vi "Autonomous Independent.vi"   [LabVIEW 2017]
doc: "This VI is called when autonomous begins, and will automatically be terminated when autonomous ends. You can carry out timed or sensor driven robot movement independently without needing to return to the caller."
uses:
  <vilib>/Rock Robotics/WPI/Utilities/WPI_GetSetVariantRefNum.vi
  <vilib>/Rock Robotics/Network Tables/NT Read Number.vi
  <vilib>/Rock Robotics/Network Tables/NT Write Numeric Array.vi
  <vilib>/Rock Robotics/Network Tables/NT Read Boolean.vi
  <vilib>/Rock Robotics/Network Tables/NT Write String.vi
  Robot Global Data.vi
  <vilib>/Rock Robotics/WPI/RobotDrive/WPI_RobotDriveArcadeDrive_Standard(NoSaturation).vi
  <vilib>/Rock Robotics/WPI/ThirdParty/Sensors/ADIS16448 IMU/ADIS16448_IMU.lvlib
panel:
  # "Be sure to right-click and choose Data Operations>>Make Current Value default if you want to save the array values with the VI"
types:
  T1 = typedef "WPI_JoystickDevRef.ctl" = cluster{"Device":T2}
  T2 = typedef "WPI_JoystickDeviceEnum.ctl" = enum16{"USB 0", "USB 1", "USB 2", "USB 3", "USB 4", "USB 5"}
  T3 = typedef "WPI_EncoderDevRef.ctl" = cluster{"DevStatus":errorcluster, "EncoderIndex":T4, "CounterIndex":T5, "DistancePerCount":dbl, "Decoding Type":T6}
  T4 = typedef "FPGA_EncoderIdx.ctl" = enum8{"Enc 0", "Enc 1", "Enc 2", "Enc 3", "Enc 4", "Enc 5", "Enc 6", "Enc 7", "Invalid"}
  T5 = typedef "FPGA_CounterCtrSystemIndex.ctl" = enum8{"Ctr 0", "Ctr 1", "Ctr 2", "Ctr 3", "Ctr 4", "Ctr 5", "Ctr 6", "Ctr 7", "Invalid"}
  T6 = typedef "WPI_EncoderType.ctl" = enum16{"1x", "2x", "4x"}
  T7 = typedef "ADIS16448_IMU.lvlib/ADI_IMU_ADIS16448_IMUDevRef.ctl" = cluster{"DevStatus":errorcluster, "Handle":i32, "SPI Bus":T8, "Device Found":bool, "Device Ready":bool, "Yaw Axis":enum16{"X", "Y", "Z"}, "AHRS Algorithm":enum16{"Complementary", "Madgwick"}, "Serial":u16, "Lot ID 2":u16, "Lot ID 1":u16, "Bytes Per Sample":u16, "Calibrate On Open?":bool}
  T8 = typedef "spi_bus.ctl" = enum16{"SPI On-Board, CS0", "SPI On-Board, CS1", "SPI On-Board, CS2", "SPI On-Board, CS3", "SPI MXP", "Invalid"}
  T9 = typedef "WPI_PotentiometerDevRef.ctl" = cluster{"DevStatus":errorcluster, "Analog Channel":T10, "Invert Output":bool}
  T10 = typedef "FPGA_AIChannel.ctl" = enum8{"AI 0", "AI 1", "AI 2", "AI 3", "AI MXP 0", "AI MXP 1", "AI MXP 2", "AI MXP 3", "Invalid"}
  T11 = typedef "WPI_RobotDriveDevRef.ctl" = cluster{"DevStatus":errorcluster, "Motors[]":T12[], "Square Inputs":bool, "Max Output":dbl}
  T12 = typedef "WPI_MotorControlDeviceRef.ctl" = cluster{"DeviceStatus":errorcluster, "Type":T13, "PWM":cluster{"PWM Channel":T14, "DeadBand":T15}, "CAN":cluster{"Device Number":u8, "SetOutput VI Ref":variant, "GetOutput VI Ref":variant, "Enable VI Ref":variant, "Disable VI Ref":variant, "Data":variant}, "Invert":bool, "DIO PWM":cluster{"PWM \"Enable\" Channel":T14, "DIOChannel":T16, "PWM Rate":dbl}}
  T13 = typedef "WPI_MotorControlType.ctl" = enum16{"PWM", "CAN", "DIO PWM"}
  T14 = typedef "FPGA_DIOPWMChannel.ctl" = enum8{"PWM 0", "PWM 1", "PWM 2", "PWM 3", "PWM 4", "PWM 5", "PWM 6", "PWM 7", "PWM 8", "PWM 9", "PWM MXP 0", "PWM MXP 1", "PWM MXP 2", "PWM MXP 3", "PWM MXP 4", "PWM MXP 5", "PWM MXP 6", "PWM MXP 7", "PWM MXP 8", "PWM MXP 9", "Invalid"}
  T15 = typedef "WPI_PWMDeadband.ctl" = cluster{"Name":string, "maxPositivePwm":i32, "minPositivePwm":i32, "centerPwm":i32, "maxNegativePwm":i32, "minNegativePwm":i32, "angularRange":u16}
  T16 = typedef "FPGA_DIOChannel.ctl" = enum8{"DIO 0", "DIO 1", "DIO 2", "DIO 3", "DIO 4", "DIO 5", "DIO 6", "DIO 7", "DIO 8", "DIO 9", "DIO MXP 0", "DIO MXP 1", "DIO MXP 2", "DIO MXP 3", "DIO MXP 4", "DIO MXP 5", "DIO MXP 6", "DIO MXP 7", "DIO MXP 8", "DIO MXP 9", "DIO MXP 10", "DIO MXP 11", "DIO MXP 12", "DIO MXP 13", "DIO MXP 14", "DIO MXP 15", "SPI Port CS1", "SPI Port CS2", "SPI Port CS3", "SPI Port MISO", "SPI Port MOSI", "Invalid"}
  T17 = cluster{"X Angle":dbl, "Y Angle":dbl, "Z Angle":dbl}
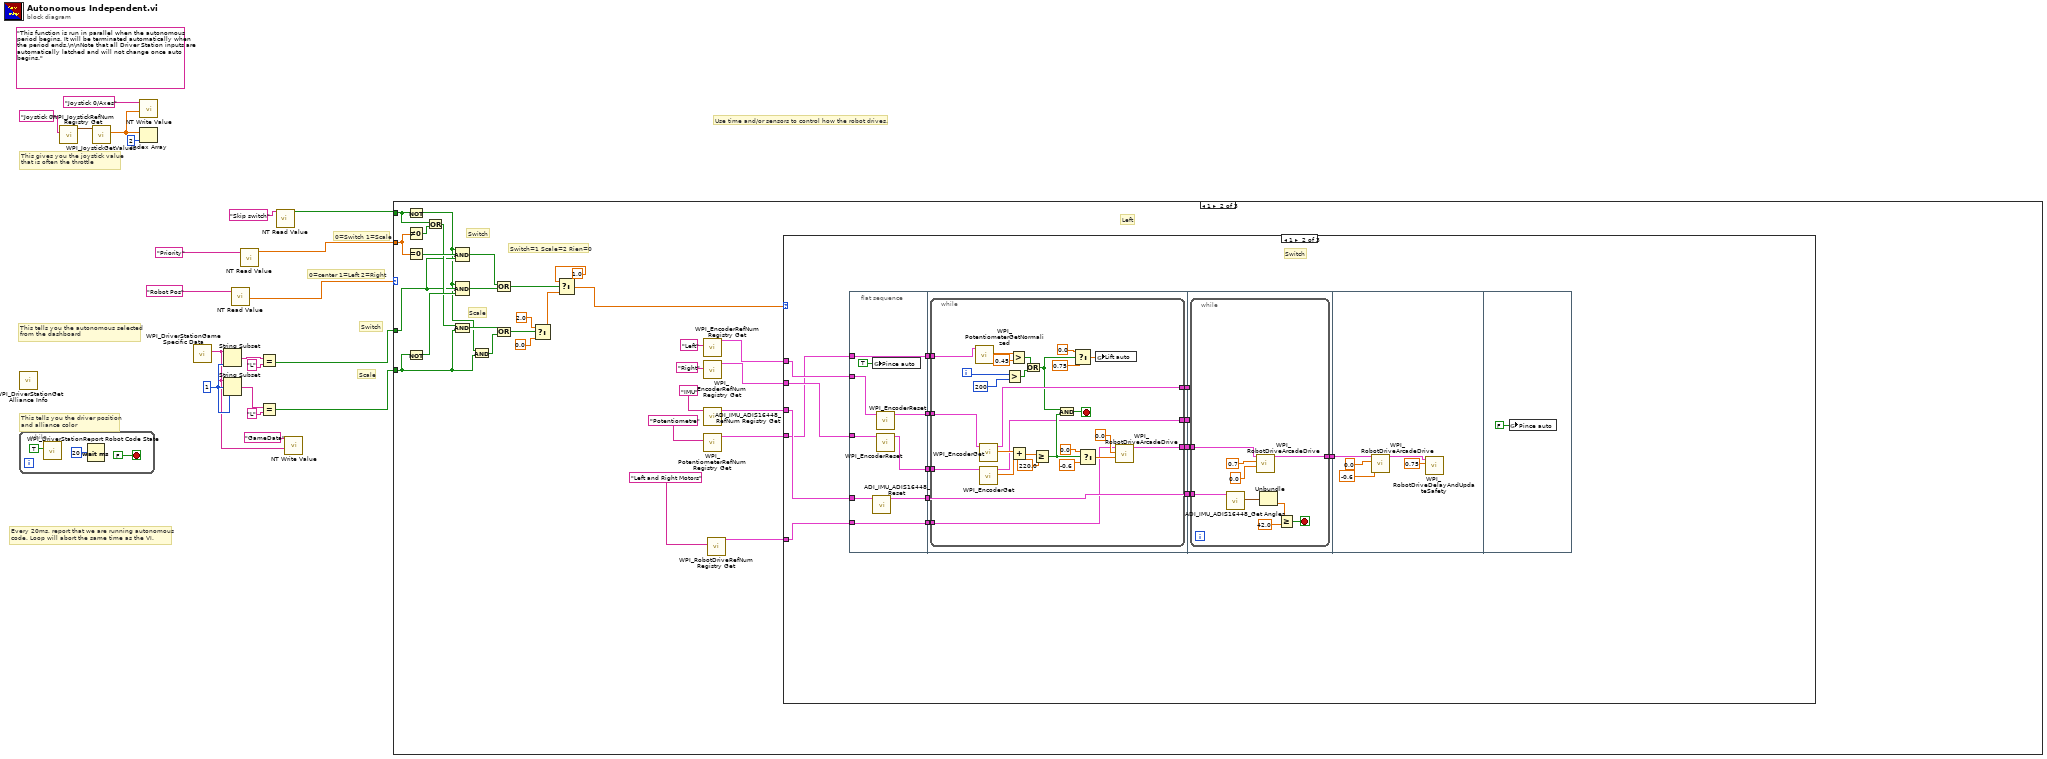
[diagram p0: block diagram]
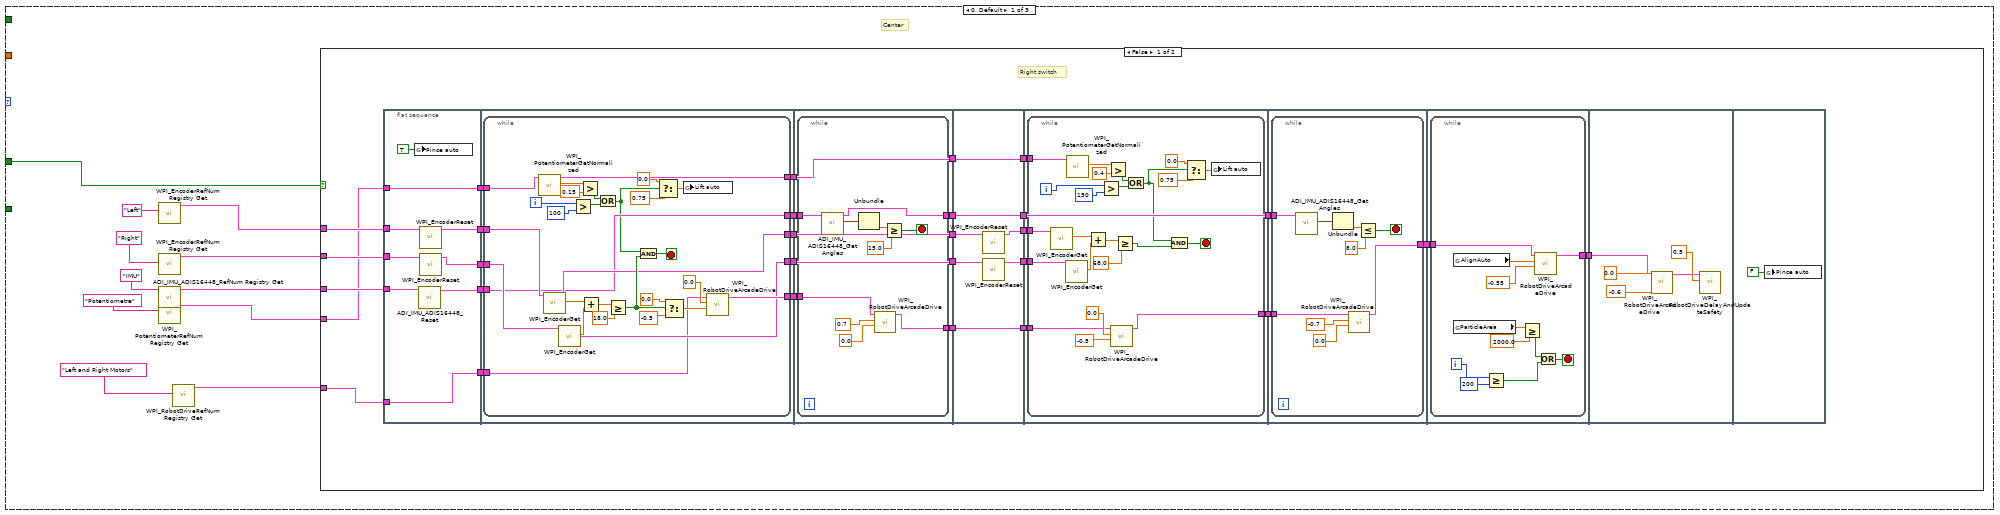
[diagram p2: hidden frame]
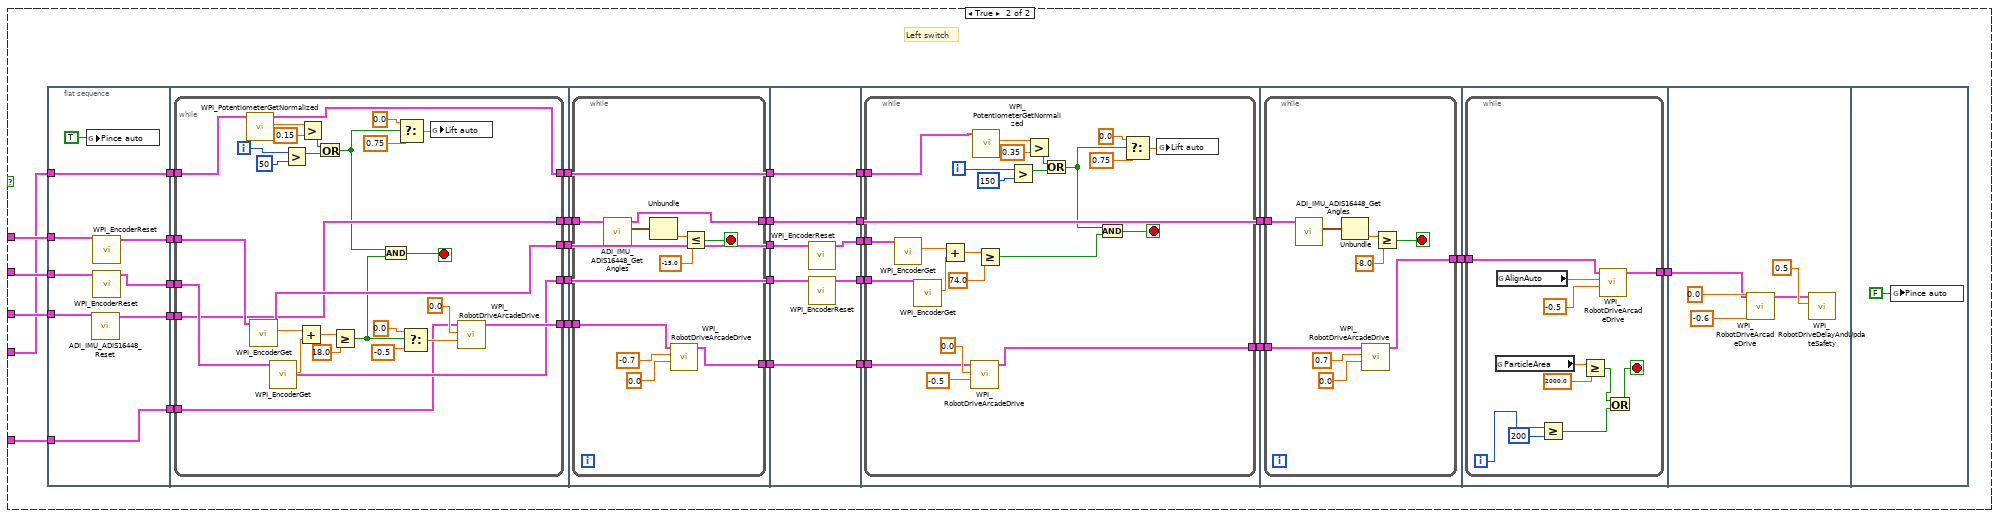
[diagram p3: hidden frame]
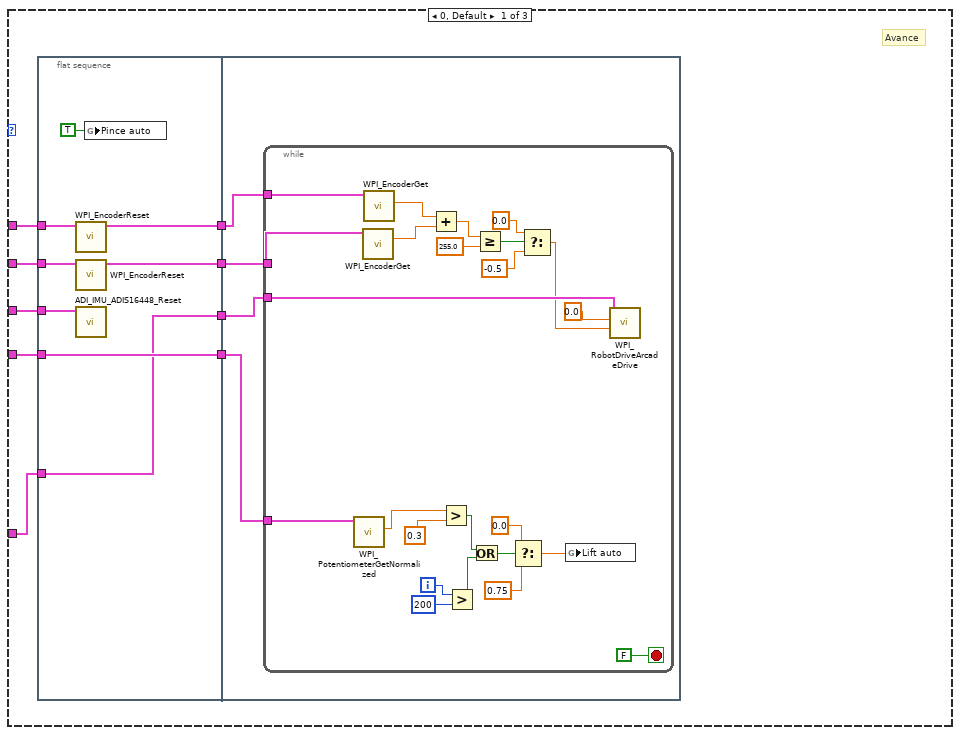
[diagram p4: hidden frame]
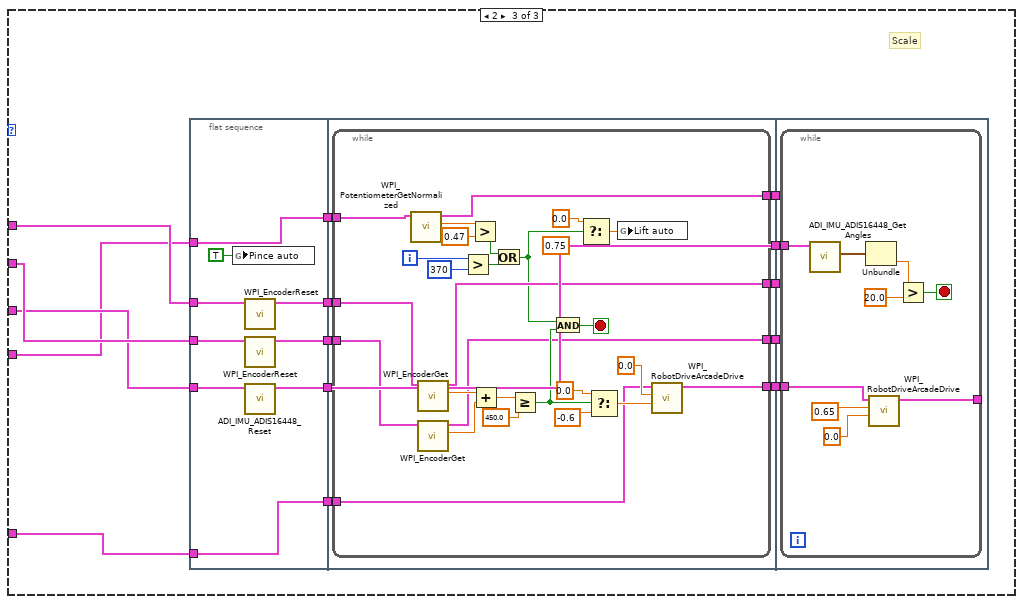
[diagram p5: hidden frame]
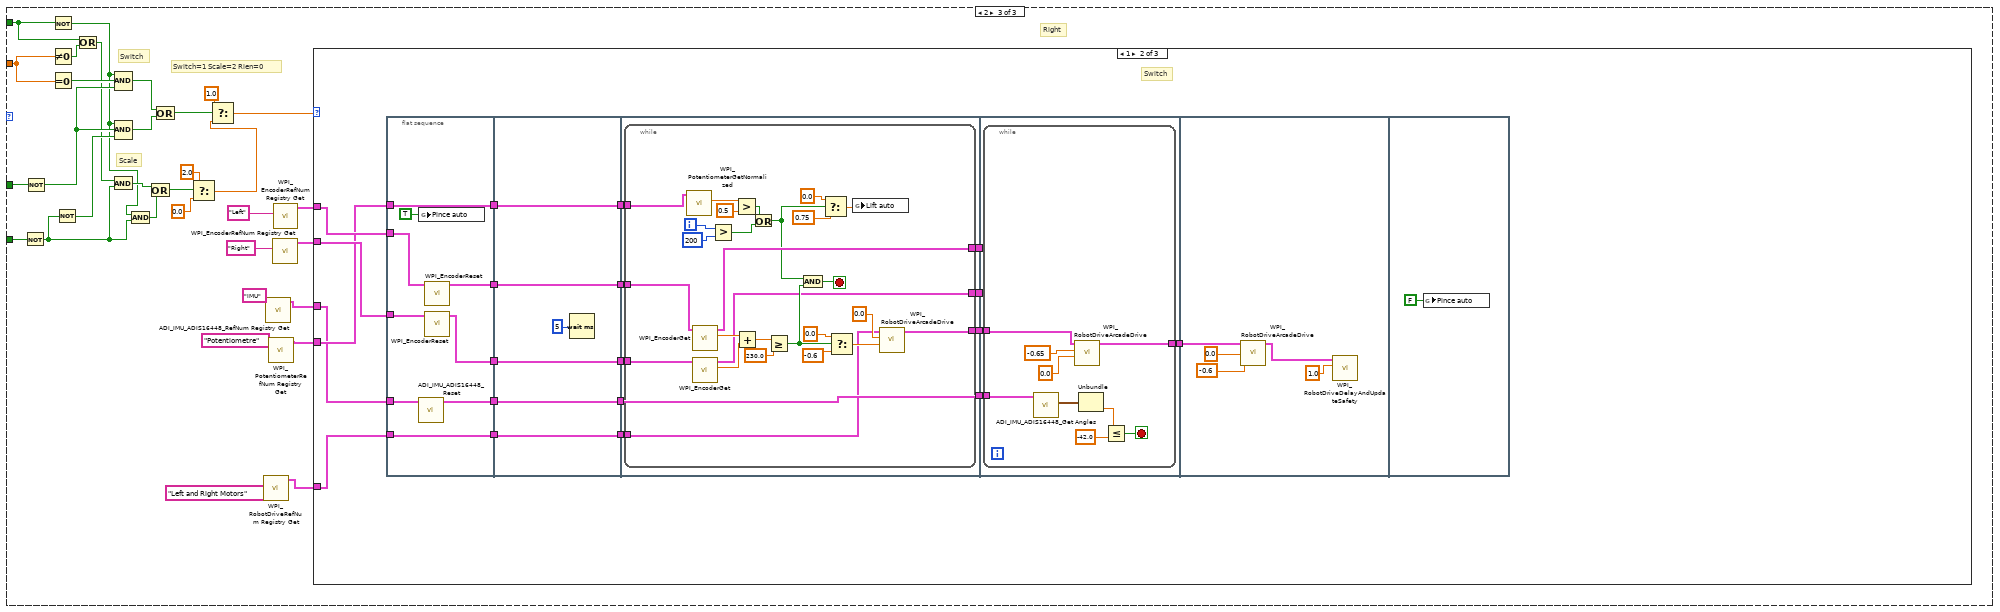
[diagram p6: hidden frame]
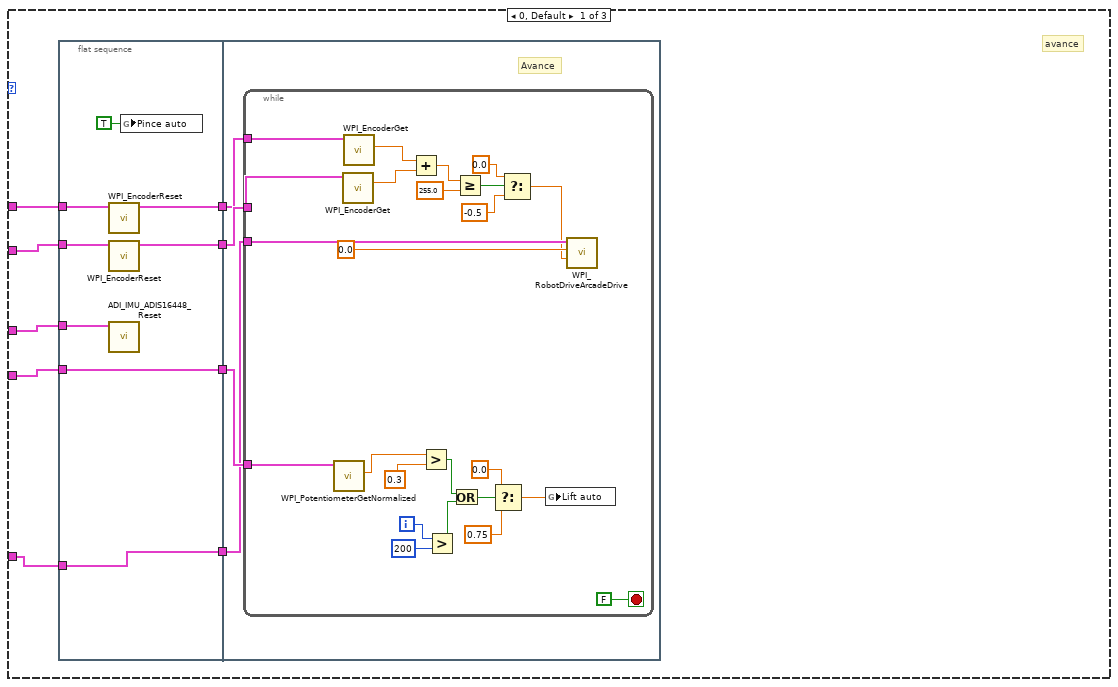
[diagram p7: hidden frame]
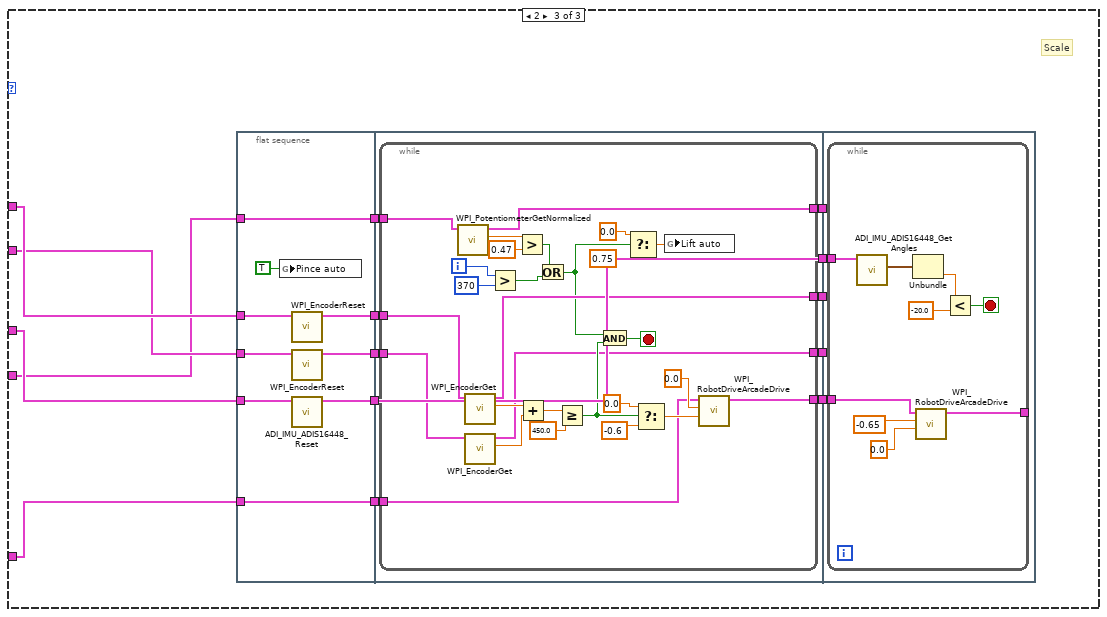
[diagram p8: hidden frame]
diagram:
  w13 = 1 ("offset (0)")
  (unwired) "This function is run in parallel when the autonomous period begins. It will be terminated automatically when the period ends.\n\nNote that all Driver Station inputs are automatically latched and will not change once auto begins."
  # "Scale"
  # "Switch"
  # "0=Switch 1=Scale"
  # "0=center 1=Left 2=Right"
  # "This tells you the autonomous selected\nfrom the dashboard"
  # "Every 20ms, report that we are running autonomous\ncode. Loop will abort the same time as the VI."
  # "This gives you the joystick value\nthat is often the throttle"
  # "Use time and/or sensors to control how the robot drives."
  # "This tells you the driver position\nand alliance color"
  n1 = while {
    stop <- FALSE stop-if-true
    n2 = call <vilib>:"WPI_DriverStationReport Robot Code State.vi"("Autonomous"=TRUE) -> ()  [unwired: 10 in, 1 out]
    n3 = Wait (ms)(milliseconds to wait=u32 20) -> ()  [unwired: 1 out]
  }
  n4 = call <vilib>:"WPI_DriverStationGet Alliance Info.vi"() -> ()  [unwired: 12 out]
  n5 = call <vilib>:"WPI_JoystickRefNum Registry Get.vi"("refnum name"="Joystick 0") -> ("JoystickDevRef"=w19:T1)  [unwired: 1 in, 9 out]
  n6 = call <vilib>:"WPI_JoystickGetValues.vi"("JoystickDevRef"=w19) -> ("Axes"=w15:dbl[])  [unwired: 6 in, 4 out]
  n7 = call-poly <vilib>:"NT Write Value.vi"("Numeric Array"=w15, "Name"="Joystick 0/Axes") -> ()  [unwired: 9 in, 1 out]
  n8 = Index Array(array=w15, index=2) -> ()  [unwired: 1 out]
  n9 = call <vilib>:"WPI_DriverStationGame Specific Data.vi"() -> ("Game Specific Data"=w2:string)  [unwired: 11 in]
  n10 = String Subset(string=w2, length (rest)=w13) -> (substring=w12:string)  [unwired: 1 in]
  n11 = String Subset(string=w2, offset (0)=w13, length (rest)=w13) -> (substring=w9:string)
  n12 = call-poly <vilib>:"NT Read Value.vi"("Name"="Robot Pos") -> ("Numeric"=w16:dbl)  [unwired: 9 in, 1 out]
  n13 = call-poly <vilib>:"NT Read Value.vi"("Name"="Priority") -> ("Numeric"=w5:dbl)  [unwired: 9 in, 1 out]
  n14 = Equal?(x=w12, y="L") -> (x = y?=w8:bool)
  n15 = Equal?(x=w9, y="L") -> (x = y?=w7:bool)
  n16 = call-poly <vilib>:"NT Read Value.vi"("Name"="Skip switch") -> ("Boolean"=w3:bool)  [unwired: 9 in, 1 out]
  n17 = call-poly <vilib>:"NT Write Value.vi"("String"=w2, "Name"="GameData") -> ()  [unwired: 9 in, 1 out]
  n18 = case shown="1" w16 {
    tunnel: w8 -> [w34 w360 w596]
    tunnel: w7 -> [_ w358 w597]
    tunnel: w5 -> [_ w372 w606]
    tunnel: w3 -> [_ w373 w607]
    frame 0, Default {
      # "Center"
      n19 = call <vilib>:"WPI_EncoderRefNum Registry Get.vi"("refnum name"="Left") -> ("EncoderDevRef"=w25:T3)  [unwired: 9 in, 1 out]
      n20 = call <vilib>:"WPI_EncoderRefNum Registry Get.vi"("refnum name"="Right") -> ("EncoderDevRef"=w26:T3)  [unwired: 9 in, 1 out]
      n21 = call <vilib>:"ADI_IMU_ADIS16448_RefNum Registry Get.vi"("refnum name"="IMU") -> ("ADI IMU DevRef"=w27:T7)  [unwired: 9 in, 1 out]
      n22 = call <vilib>:"WPI_PotentiometerRefNum Registry Get.vi"("refnum name"="Potentiometre") -> ("PotDevRef"=w28:T9)  [unwired: 9 in, 1 out]
      n23 = call <vilib>:"WPI_RobotDriveRefNum Registry Get.vi"("refnum name"="Left and Right Motors") -> ("RobotDriveDevRef"=w24:T11)  [unwired: 9 in, 1 out]
      n24 = case shown="False" w34 {
        tunnel: w28 -> [w40 w201]
        tunnel: w27 -> [w42 w203]
        tunnel: w26 -> [w43 w204]
        tunnel: w25 -> [w44 w205]
        tunnel: w24 -> [w38 w199]
        frame False {
          # "Right switch"
          n25 = flat-sequence {
            tunnel: [w71] -> w63
            tunnel: [w70] -> w62
            tunnel: [w69] -> w61
            tunnel: w44 -> [w68]
            tunnel: w43 -> [w67]
            tunnel: w42 -> [w66]
            tunnel: [w65] -> w41
            tunnel: w40 -> [w65]
            tunnel: [w64] -> w39
            tunnel: w38 -> [w64]
            tunnel: [w82] -> w60
            tunnel: [w81] -> w59
            tunnel: [w80] -> w58
            tunnel: w63 -> [w79]
            tunnel: w62 -> [w78]
            tunnel: w61 -> [w77]
            tunnel: [w76] -> w57
            tunnel: w41 -> [w75]
            tunnel: w39 -> [w74]
            tunnel: [w73] -> w35
            tunnel: [w118] -> w56
            tunnel: [w117] -> w55
            tunnel: w60 -> [w116]
            tunnel: w59 -> [w115]
            tunnel: [w115] -> w54
            tunnel: w58 -> [w114]
            tunnel: [w114] -> w53
            tunnel: w57 -> [w113]
            tunnel: [w112] -> w36
            tunnel: w35 -> [w112]
            tunnel: [w135] -> w52
            tunnel: [w134] -> w51
            tunnel: w56 -> [w133]
            tunnel: [w133] -> w50
            tunnel: [w132] -> w49
            tunnel: w55 -> [w132]
            tunnel: w54 -> [w131]
            tunnel: w53 -> [w130]
            tunnel: [w129] -> w37
            tunnel: w36 -> [w129]
            tunnel: [w141] -> w48
            tunnel: w52 -> [w140]
            tunnel: w51 -> [w139]
            tunnel: w50 -> [w138]
            tunnel: [w138] -> w47
            tunnel: w49 -> [w137]
            tunnel: w37 -> [w136]
            tunnel: [w167] -> w46
            tunnel: w48 -> [w166]
            tunnel: w47 -> [w165]
            tunnel: [w178] -> w45
            tunnel: w46 -> [w177]
            tunnel: w45 -> [w190]
            frame #0 {
              n26 = global write "Robot Global Data.vi" "Pince auto"(TRUE ("Pince auto")) -> ()
              n27 = call <vilib>:"ADI_IMU_ADIS16448_Reset.vi"("ADI IMU DevRef"=w66) -> ("ADI IMU DevRef Out"=w69:T7)  [unwired: 9 in, 1 out]
              n28 = call <vilib>:"WPI_EncoderReset.vi"("EncoderDevRef"=w68) -> ("EncoderDevRef"=w71:T3)  [unwired: 9 in, 1 out]
              n29 = call <vilib>:"WPI_EncoderReset.vi"("EncoderDevRef"=w67) -> ("EncoderDevRef"=w70:T3)  [unwired: 9 in, 1 out]
            }
            frame #1 {
              n30 = while {
                tunnel: [w96] -> w82
                tunnel: [w95] -> w81
                tunnel: [w94] -> w80
                tunnel: w79 -> [w93]
                tunnel: w78 -> [w92]
                tunnel: w77 -> [w91]
                tunnel: [w91] -> w76
                tunnel: w75 -> [w90]
                tunnel: w74 -> [w89]
                tunnel: [w83] -> w73
                i -> [w85]
                stop <- w98 stop-if-true
                n31 = call <vilib>:"WPI_PotentiometerGetNormalized.vi"("PotDevRef"=w90) -> ("Normalized Value"=w111:dbl, "PotDevRef"=w83:T9)  [unwired: 8 in, 1 out]
                n32 = call <vilib>:"WPI_EncoderGet.vi"("EncoderDevRef"=w93) -> ("Distance"=w106:dbl, "EncoderDevRef"=w94:T3)  [unwired: 5 in, 4 out]
                n33 = call <vilib>:"WPI_EncoderGet.vi"("EncoderDevRef"=w92) -> ("Distance"=w105:dbl, "EncoderDevRef"=w95:T3)  [unwired: 5 in, 4 out]
                n34 = Greater?(x=w85, y=100) -> (0:w86:bool)
                n35 = Greater?(x=w111, y=0.15) -> (0:w88:bool)
                n36 = Add(x=w106, y=w105) -> (x+y=w104:dbl)
                n37 = Or(x=w88, y=w86) -> (x .or. y?=w87:bool)
                n38 = Greater Or Equal?(x=w104, y=18.0) -> (x >= y?=w97:bool)
                n39 = And(x=w87, y=w97) -> (x .and. y?=w98:bool)
                n40 = Select(t=0.0, s=w87, f=0.75) -> (s? t:f=w107:dbl)
                n41 = Select(t=0.0, s=w97, f=-0.5) -> (s? t:f=w99:dbl)
                n42 = global write "Robot Global Data.vi" "Lift auto"(w107) -> ()
                n43 = call-poly <vilib>:"WPI_RobotDriveArcadeDrive.vi"("Y axis value"=w99, "X axis value"=0.0, "RobotDriveDevRef"=w89) -> ("RobotDriveDevRef"=w96:T11)  [unwired: 6 in, 2 out]
              }
            }
            frame #2 {
              n44 = while {
                tunnel: [w122] -> w118
                tunnel: [w121] -> w117
                tunnel: w116 -> [w120]
                tunnel: w113 -> [w119]
                stop <- w125 stop-if-true
                n45 = call <vilib>:"ADI_IMU_ADIS16448_Get Angles.vi"("ADI IMU DevRef"=w119) -> ("IMU Angles Out"=w126:T17, "ADI IMU DevRef Out"=w122:T7)  [unwired: 7 in, 2 out]
                n46 = Unbundle(w126) -> ("Z Angle"=w128:dbl)  [unwired: 2 out]
                n47 = call-poly <vilib>:"WPI_RobotDriveArcadeDrive.vi"("Y axis value"=0.0, "X axis value"=0.7, "RobotDriveDevRef"=w120) -> ("RobotDriveDevRef"=w121:T11)  [unwired: 6 in, 2 out]
                n48 = Greater Or Equal?(x=w128, y=15.0) -> (x >= y?=w125:bool)
              }
            }
            frame #3 {
              n49 = call <vilib>:"WPI_EncoderReset.vi"("EncoderDevRef"=w130) -> ("EncoderDevRef"=w135:T3)  [unwired: 9 in, 1 out]
              n50 = call <vilib>:"WPI_EncoderReset.vi"("EncoderDevRef"=w131) -> ("EncoderDevRef"=w134:T3)  [unwired: 9 in, 1 out]
            }
            frame #4 {
              n51 = while {
                tunnel: [w158] -> w141
                tunnel: w140 -> [w157]
                tunnel: w139 -> [w156]
                tunnel: w137 -> [w155]
                tunnel: w136 -> [w142]
                i -> [w143]
                stop <- w146 stop-if-true
                n52 = call <vilib>:"WPI_EncoderGet.vi"("EncoderDevRef"=w157) -> ("Distance"=w164:dbl)  [unwired: 5 in, 5 out]
                n53 = call <vilib>:"WPI_EncoderGet.vi"("EncoderDevRef"=w156) -> ("Distance"=w163:dbl)  [unwired: 5 in, 5 out]
                n54 = call <vilib>:"WPI_PotentiometerGetNormalized.vi"("PotDevRef"=w142) -> ("Normalized Value"=w154:dbl)  [unwired: 8 in, 2 out]
                n55 = Add(x=w164, y=w163) -> (x+y=w162:dbl)
                n56 = Greater?(x=w143, y=150) -> (0:w148:bool)
                n57 = Greater?(x=w154, y=0.4) -> (0:w149:bool)
                n58 = call-poly <vilib>:"WPI_RobotDriveArcadeDrive.vi"("Y axis value"=-0.5 ("f"), "X axis value"=0.0, "RobotDriveDevRef"=w155) -> ("RobotDriveDevRef"=w158:T11)  [unwired: 6 in, 2 out]
                n59 = Greater Or Equal?(x=w162, y=68.0) -> (x >= y?=w145:bool)
                n60 = Or(x=w149, y=w148) -> (x .or. y?=w144:bool)
                n61 = And(x=w144, y=w145) -> (x .and. y?=w146:bool)
                n62 = Select(t=0.0, s=w144, f=0.75) -> (s? t:f=w150:dbl)
                n63 = global write "Robot Global Data.vi" "Lift auto"(w150) -> ()
              }
            }
            frame #5 {
              n64 = while {
                tunnel: [w170] -> w167
                tunnel: w166 -> [w169]
                tunnel: w165 -> [w168]
                stop <- w173 stop-if-true
                n65 = call <vilib>:"ADI_IMU_ADIS16448_Get Angles.vi"("ADI IMU DevRef"=w168) -> ("IMU Angles Out"=w174:T17)  [unwired: 7 in, 3 out]
                n66 = Unbundle(w174) -> ("Z Angle"=w176:dbl)  [unwired: 2 out]
                n67 = call-poly <vilib>:"WPI_RobotDriveArcadeDrive.vi"("Y axis value"=0.0, "X axis value"=-0.7, "RobotDriveDevRef"=w169) -> ("RobotDriveDevRef"=w170:T11)  [unwired: 6 in, 2 out]
                n68 = Less Or Equal?(x=w176, y=8.0) -> (x <= y?=w173:bool)
              }
            }
            frame #6 {
              n69 = while {
                tunnel: [w185] -> w178
                tunnel: w177 -> [w184]
                i -> [w183]
                stop <- w181 stop-if-true
                n70 = global read "Robot Global Data.vi" "ParticleArea"() -> (w187:dbl)
                n71 = global read "Robot Global Data.vi" "AlignAuto"() -> (w189:dbl)
                n72 = Greater Or Equal?(x=w183, y=200) -> (x >= y?=w179:bool)
                n73 = Greater Or Equal?(x=w187, y=2000.0) -> (x >= y?=w180:bool)
                n74 = call-poly <vilib>:"WPI_RobotDriveArcadeDrive.vi"("Y axis value"=-0.55, "X axis value"=w189, "RobotDriveDevRef"=w184) -> ("RobotDriveDevRef"=w185:T11)  [unwired: 6 in, 2 out]
                n75 = Or(x=w180, y=w179) -> (x .or. y?=w181:bool)
              }
            }
            frame #7 {
              n76 = call-poly <vilib>:"WPI_RobotDriveArcadeDrive.vi"("Y axis value"=-0.6, "X axis value"=0.0, "RobotDriveDevRef"=w190) -> ("RobotDriveDevRef"=w191:T11)  [unwired: 6 in, 2 out]
              n77 = call <vilib>:"WPI_RobotDriveDelayAndUpdateSafety.vi"("Delay (s)"=0.5, "RobotDriveDevRef"=w191) -> ()  [unwired: 8 in, 2 out]
            }
            frame #8 {
              n78 = global write "Robot Global Data.vi" "Pince auto"(FALSE ("Pince auto")) -> ()
            }
          }
        }
        frame True {
          # "Left switch"
          n79 = flat-sequence {
            tunnel: [w232] -> w224
            tunnel: [w231] -> w223
            tunnel: [w230] -> w222
            tunnel: w205 -> [w229]
            tunnel: w204 -> [w228]
            tunnel: w203 -> [w227]
            tunnel: [w226] -> w202
            tunnel: w201 -> [w226]
            tunnel: [w225] -> w200
            tunnel: w199 -> [w225]
            tunnel: [w243] -> w221
            tunnel: [w242] -> w220
            tunnel: [w241] -> w219
            tunnel: w224 -> [w240]
            tunnel: w223 -> [w239]
            tunnel: w222 -> [w238]
            tunnel: [w237] -> w218
            tunnel: w202 -> [w236]
            tunnel: w200 -> [w235]
            tunnel: [w234] -> w198
            tunnel: [w279] -> w217
            tunnel: [w278] -> w216
            tunnel: w221 -> [w277]
            tunnel: w220 -> [w276]
            tunnel: [w276] -> w215
            tunnel: w219 -> [w275]
            tunnel: [w275] -> w214
            tunnel: w218 -> [w274]
            tunnel: w198 -> [w273]
            tunnel: [w273] -> w197
            tunnel: [w296] -> w213
            tunnel: [w295] -> w212
            tunnel: w217 -> [w294]
            tunnel: [w294] -> w211
            tunnel: [w293] -> w210
            tunnel: w216 -> [w293]
            tunnel: w215 -> [w292]
            tunnel: w214 -> [w291]
            tunnel: w197 -> [w290]
            tunnel: [w290] -> w196
            tunnel: [w302] -> w209
            tunnel: w213 -> [w301]
            tunnel: w212 -> [w300]
            tunnel: w211 -> [w299]
            tunnel: [w299] -> w208
            tunnel: w210 -> [w298]
            tunnel: w196 -> [w297]
            tunnel: [w328] -> w207
            tunnel: w209 -> [w327]
            tunnel: w208 -> [w326]
            tunnel: [w339] -> w206
            tunnel: w207 -> [w338]
            tunnel: w206 -> [w351]
            frame #0 {
              n80 = global write "Robot Global Data.vi" "Pince auto"(TRUE ("Pince auto")) -> ()
              n81 = call <vilib>:"ADI_IMU_ADIS16448_Reset.vi"("ADI IMU DevRef"=w227) -> ("ADI IMU DevRef Out"=w230:T7)  [unwired: 9 in, 1 out]
              n82 = call <vilib>:"WPI_EncoderReset.vi"("EncoderDevRef"=w229) -> ("EncoderDevRef"=w232:T3)  [unwired: 9 in, 1 out]
              n83 = call <vilib>:"WPI_EncoderReset.vi"("EncoderDevRef"=w228) -> ("EncoderDevRef"=w231:T3)  [unwired: 9 in, 1 out]
            }
            frame #1 {
              n84 = while {
                tunnel: [w264] -> w243
                tunnel: [w263] -> w242
                tunnel: [w262] -> w241
                tunnel: w240 -> [w261]
                tunnel: w239 -> [w260]
                tunnel: w238 -> [w259]
                tunnel: [w259] -> w237
                tunnel: w236 -> [w250]
                tunnel: w235 -> [w258]
                tunnel: [w249] -> w234
                i -> [w248]
                stop <- w247 stop-if-true
                n85 = call <vilib>:"WPI_PotentiometerGetNormalized.vi"("PotDevRef"=w250) -> ("Normalized Value"=w257:dbl, "PotDevRef"=w249:T9)  [unwired: 8 in, 1 out]
                n86 = call <vilib>:"WPI_EncoderGet.vi"("EncoderDevRef"=w261) -> ("Distance"=w272:dbl, "EncoderDevRef"=w262:T3)  [unwired: 5 in, 4 out]
                n87 = call <vilib>:"WPI_EncoderGet.vi"("EncoderDevRef"=w260) -> ("Distance"=w271:dbl, "EncoderDevRef"=w263:T3)  [unwired: 5 in, 4 out]
                n88 = Greater?(x=w248, y=50) -> (0:w246:bool)
                n89 = Add(x=w272, y=w271) -> (x+y=w270:dbl)
                n90 = Greater?(x=w257, y=0.15) -> (0:w252:bool)
                n91 = Or(x=w252, y=w246) -> (x .or. y?=w244:bool)
                n92 = Greater Or Equal?(x=w270, y=18.0) -> (x >= y?=w245:bool)
                n93 = And(x=w244, y=w245) -> (x .and. y?=w247:bool)
                n94 = Select(t=0.0, s=w244, f=0.75) -> (s? t:f=w253:dbl)
                n95 = Select(t=0.0, s=w245, f=-0.5) -> (s? t:f=w265:dbl)
                n96 = global write "Robot Global Data.vi" "Lift auto"(w253) -> ()
                n97 = call-poly <vilib>:"WPI_RobotDriveArcadeDrive.vi"("Y axis value"=w265, "X axis value"=0.0, "RobotDriveDevRef"=w258) -> ("RobotDriveDevRef"=w264:T11)  [unwired: 6 in, 2 out]
              }
            }
            frame #2 {
              n98 = while {
                tunnel: [w283] -> w279
                tunnel: [w282] -> w278
                tunnel: w277 -> [w281]
                tunnel: w274 -> [w280]
                stop <- w286 stop-if-true
                n99 = call <vilib>:"ADI_IMU_ADIS16448_Get Angles.vi"("ADI IMU DevRef"=w280) -> ("IMU Angles Out"=w287:T17, "ADI IMU DevRef Out"=w283:T7)  [unwired: 7 in, 2 out]
                n100 = Unbundle(w287) -> ("Z Angle"=w289:dbl)  [unwired: 2 out]
                n101 = call-poly <vilib>:"WPI_RobotDriveArcadeDrive.vi"("Y axis value"=0.0, "X axis value"=-0.7, "RobotDriveDevRef"=w281) -> ("RobotDriveDevRef"=w282:T11)  [unwired: 6 in, 2 out]
                n102 = Less Or Equal?(x=w289, y=-15.0) -> (x <= y?=w286:bool)
              }
            }
            frame #3 {
              n103 = call <vilib>:"WPI_EncoderReset.vi"("EncoderDevRef"=w291) -> ("EncoderDevRef"=w296:T3)  [unwired: 9 in, 1 out]
              n104 = call <vilib>:"WPI_EncoderReset.vi"("EncoderDevRef"=w292) -> ("EncoderDevRef"=w295:T3)  [unwired: 9 in, 1 out]
            }
            frame #4 {
              n105 = while {
                tunnel: [w319] -> w302
                tunnel: w301 -> [w318]
                tunnel: w300 -> [w317]
                tunnel: w298 -> [w316]
                tunnel: w297 -> [w304]
                i -> [w303]
                stop <- w305 stop-if-true
                n106 = call <vilib>:"WPI_EncoderGet.vi"("EncoderDevRef"=w318) -> ("Distance"=w325:dbl)  [unwired: 5 in, 5 out]
                n107 = call <vilib>:"WPI_EncoderGet.vi"("EncoderDevRef"=w317) -> ("Distance"=w324:dbl)  [unwired: 5 in, 5 out]
                n108 = Add(x=w325, y=w324) -> (x+y=w323:dbl)
                n109 = call-poly <vilib>:"WPI_RobotDriveArcadeDrive.vi"("Y axis value"=-0.5 ("f"), "X axis value"=0.0, "RobotDriveDevRef"=w316) -> ("RobotDriveDevRef"=w319:T11)  [unwired: 6 in, 2 out]
                n110 = call <vilib>:"WPI_PotentiometerGetNormalized.vi"("PotDevRef"=w304) -> ("Normalized Value"=w315:dbl)  [unwired: 8 in, 2 out]
                n111 = Greater Or Equal?(x=w323, y=74.0) -> (x >= y?=w306:bool)
                n112 = Greater?(x=w303, y=150) -> (0:w308:bool)
                n113 = Greater?(x=w315, y=0.35) -> (0:w310:bool)
                n114 = Or(x=w310, y=w308) -> (x .or. y?=w309:bool)
                n115 = And(x=w309, y=w306) -> (x .and. y?=w305:bool)
                n116 = Select(t=0.0, s=w309, f=0.75) -> (s? t:f=w311:dbl)
                n117 = global write "Robot Global Data.vi" "Lift auto"(w311) -> ()
              }
            }
            frame #5 {
              n118 = while {
                tunnel: [w331] -> w328
                tunnel: w327 -> [w330]
                tunnel: w326 -> [w329]
                stop <- w334 stop-if-true
                n119 = call <vilib>:"ADI_IMU_ADIS16448_Get Angles.vi"("ADI IMU DevRef"=w329) -> ("IMU Angles Out"=w335:T17)  [unwired: 7 in, 3 out]
                n120 = Unbundle(w335) -> ("Z Angle"=w337:dbl)  [unwired: 2 out]
                n121 = call-poly <vilib>:"WPI_RobotDriveArcadeDrive.vi"("Y axis value"=0.0, "X axis value"=0.7, "RobotDriveDevRef"=w330) -> ("RobotDriveDevRef"=w331:T11)  [unwired: 6 in, 2 out]
                n122 = Greater Or Equal?(x=w337, y=-8.0) -> (x >= y?=w334:bool)
              }
            }
            frame #6 {
              n123 = while {
                tunnel: [w346] -> w339
                tunnel: w338 -> [w345]
                i -> [w340]
                stop <- w342 stop-if-true
                n124 = global read "Robot Global Data.vi" "ParticleArea"() -> (w348:dbl)
                n125 = global read "Robot Global Data.vi" "AlignAuto"() -> (w350:dbl)
                n126 = Greater Or Equal?(x=w340, y=200) -> (x >= y?=w343:bool)
                n127 = Greater Or Equal?(x=w348, y=2000.0) -> (x >= y?=w341:bool)
                n128 = call-poly <vilib>:"WPI_RobotDriveArcadeDrive.vi"("Y axis value"=-0.5, "X axis value"=w350, "RobotDriveDevRef"=w345) -> ("RobotDriveDevRef"=w346:T11)  [unwired: 6 in, 2 out]
                n129 = Or(x=w341, y=w343) -> (x .or. y?=w342:bool)
              }
            }
            frame #7 {
              n130 = call-poly <vilib>:"WPI_RobotDriveArcadeDrive.vi"("Y axis value"=-0.6, "X axis value"=0.0, "RobotDriveDevRef"=w351) -> ("RobotDriveDevRef"=w352:T11)  [unwired: 6 in, 2 out]
              n131 = call <vilib>:"WPI_RobotDriveDelayAndUpdateSafety.vi"("Delay (s)"=0.5, "RobotDriveDevRef"=w352) -> ()  [unwired: 8 in, 2 out]
            }
            frame #8 {
              n132 = global write "Robot Global Data.vi" "Pince auto"(FALSE ("Pince auto")) -> ()
            }
          }
        }
      }
    }
    frame 1 {
      # "Switch=1 Scale=2 Rien=0"
      # "Scale"
      # "Switch"
      # "Left"
      n133 = Not(x=w373) -> (.not. x?=w357:bool)
      n134 = Not Equal To 0?(x=w372) -> (x != 0?=w381:bool)
      n135 = Equal To 0?(x=w372) -> (x = 0?=w383:bool)
      n136 = Not(x=w358) -> (.not. x?=w384:bool)
      n137 = Or(x=w373, y=w381) -> (x .or. y?=w361:bool)
      n138 = Compound Arithmetic op=AND(w357, w383, w360) -> (w386:bool)
      n139 = Compound Arithmetic op=AND(w357, w360, w384) -> (w385:bool)
      n140 = Compound Arithmetic op=AND(w361, w358) -> (w382:bool)
      n141 = And(x=w357, y=w358) -> (x .and. y?=w359:bool)
      n142 = Compound Arithmetic op=OR(w386, w385) -> (w380:bool)
      n143 = Compound Arithmetic op=OR(w382, w359) -> (w378:bool)
      n144 = Select(t=2.0, s=w378, f=0.0) -> (s? t:f=w376:dbl)
      n145 = Select(t=1.0, s=w380, f=w376) -> (s? t:f=w374:dbl)
      n146 = call <vilib>:"WPI_EncoderRefNum Registry Get.vi"("refnum name"="Left") -> ("EncoderDevRef"=w369:T3)  [unwired: 9 in, 1 out]
      n147 = call <vilib>:"WPI_EncoderRefNum Registry Get.vi"("refnum name"="Right") -> ("EncoderDevRef"=w370:T3)  [unwired: 9 in, 1 out]
      n148 = call <vilib>:"ADI_IMU_ADIS16448_RefNum Registry Get.vi"("refnum name"="IMU") -> ("ADI IMU DevRef"=w371:T7)  [unwired: 9 in, 1 out]
      n149 = call <vilib>:"WPI_PotentiometerRefNum Registry Get.vi"("refnum name"="Potentiometre") -> ("PotDevRef"=w367:T9)  [unwired: 9 in, 1 out]
      n150 = call <vilib>:"WPI_RobotDriveRefNum Registry Get.vi"("refnum name"="Left and Right Motors") -> ("RobotDriveDevRef"=w368:T11)  [unwired: 9 in, 1 out]
      n151 = case shown="1" w374 {
        tunnel: w371 -> [w395 w437 w513]
        tunnel: w370 -> [w394 w438 w514]
        tunnel: w369 -> [w393 w439 w515]
        tunnel: w368 -> [w389 w433 w509]
        tunnel: w367 -> [w392 w435 w511]
        frame 0, Default {
          # "Avance"
          n152 = flat-sequence {
            tunnel: w395 -> [w403]
            tunnel: w394 -> [w402]
            tunnel: w393 -> [w401]
            tunnel: w392 -> [w397]
            tunnel: [w400] -> w391
            tunnel: [w399] -> w390
            tunnel: w389 -> [w396]
            tunnel: [w397] -> w388
            tunnel: [w396] -> w387
            tunnel: w391 -> [w406]
            tunnel: w390 -> [w405]
            tunnel: w388 -> [w407]
            tunnel: w387 -> [w404]
            frame #0 {
              n153 = call <vilib>:"WPI_EncoderReset.vi"("EncoderDevRef"=w401) -> ("EncoderDevRef"=w400:T3)  [unwired: 9 in, 1 out]
              n154 = call <vilib>:"WPI_EncoderReset.vi"("EncoderDevRef"=w402) -> ("EncoderDevRef"=w399:T3)  [unwired: 9 in, 1 out]
              n155 = call <vilib>:"ADI_IMU_ADIS16448_Reset.vi"("ADI IMU DevRef"=w403) -> ()  [unwired: 9 in, 2 out]
              n156 = global write "Robot Global Data.vi" "Pince auto"(TRUE ("Pince auto")) -> ()
            }
            frame #1 {
              n157 = while {
                tunnel: w407 -> [w431]
                tunnel: w406 -> [w430]
                tunnel: w405 -> [w429]
                tunnel: w404 -> [w428]
                i -> [w409]
                stop <- FALSE stop-if-true
                n158 = call <vilib>:"WPI_PotentiometerGetNormalized.vi"("PotDevRef"=w431) -> ("Normalized Value"=w418:dbl)  [unwired: 8 in, 2 out]
                n159 = call <vilib>:"WPI_EncoderGet.vi"("EncoderDevRef"=w429) -> ("Distance"=w426:dbl)  [unwired: 5 in, 5 out]
                n160 = call <vilib>:"WPI_EncoderGet.vi"("EncoderDevRef"=w430) -> ("Distance"=w427:dbl)  [unwired: 5 in, 5 out]
                n161 = Add(x=w427, y=w426) -> (x+y=w425:dbl)
                n162 = Greater?(x=w418, y=0.3) -> (0:w415:bool)
                n163 = Greater?(x=w409, y=200) -> (0:w416:bool)
                n164 = Or(x=w415, y=w416) -> (x .or. y?=w414:bool)
                n165 = Greater Or Equal?(x=w425, y=255.0) -> (x >= y?=w422:bool)
                n166 = Select(t=0.0 ("Lift auto"), s=w414, f=0.75 ("Lift auto")) -> (s? t:f=w412:dbl)
                n167 = Select(t=0.0, s=w422, f=-0.5 ("Y axis value")) -> (s? t:f=w420:dbl)
                n168 = global write "Robot Global Data.vi" "Lift auto"(w412) -> ()
                n169 = call-poly <vilib>:"WPI_RobotDriveArcadeDrive.vi"("Y axis value"=w420, "X axis value"=0.0, "RobotDriveDevRef"=w428) -> ()  [unwired: 6 in, 3 out]
              }
            }
          }
        }
        frame 1 {
          # "Switch"
          n170 = flat-sequence {
            tunnel: [w454] -> w446
            tunnel: [w453] -> w445
            tunnel: [w452] -> w444
            tunnel: w439 -> [w451]
            tunnel: w438 -> [w450]
            tunnel: w437 -> [w449]
            tunnel: [w448] -> w436
            tunnel: w435 -> [w448]
            tunnel: [w447] -> w434
            tunnel: w433 -> [w447]
            tunnel: w446 -> [w463]
            tunnel: w445 -> [w462]
            tunnel: [w461] -> w443
            tunnel: w444 -> [w461]
            tunnel: [w460] -> w442
            tunnel: [w459] -> w441
            tunnel: [w458] -> w440
            tunnel: w436 -> [w457]
            tunnel: w434 -> [w456]
            tunnel: w443 -> [w493]
            tunnel: w442 -> [w492]
            tunnel: w441 -> [_]
            tunnel: w440 -> [_]
            tunnel: [w491] -> w432
            tunnel: w432 -> [w507]
            frame #0 {
              n171 = global write "Robot Global Data.vi" "Pince auto"(TRUE ("Pince auto")) -> ()
              n172 = call <vilib>:"ADI_IMU_ADIS16448_Reset.vi"("ADI IMU DevRef"=w449) -> ("ADI IMU DevRef Out"=w452:T7)  [unwired: 9 in, 1 out]
              n173 = call <vilib>:"WPI_EncoderReset.vi"("EncoderDevRef"=w451) -> ("EncoderDevRef"=w454:T3)  [unwired: 9 in, 1 out]
              n174 = call <vilib>:"WPI_EncoderReset.vi"("EncoderDevRef"=w450) -> ("EncoderDevRef"=w453:T3)  [unwired: 9 in, 1 out]
            }
            frame #1 {
              n175 = while {
                tunnel: w463 -> [w475]
                tunnel: w462 -> [w474]
                tunnel: [w473] -> w459
                tunnel: [w472] -> w458
                tunnel: [w471] -> w460
                tunnel: w457 -> [w470]
                tunnel: w456 -> [w469]
                i -> [w468]
                stop <- w477 stop-if-true
                n176 = call <vilib>:"WPI_PotentiometerGetNormalized.vi"("PotDevRef"=w470) -> ("Normalized Value"=w490:dbl)  [unwired: 8 in, 2 out]
                n177 = call <vilib>:"WPI_EncoderGet.vi"("EncoderDevRef"=w475) -> ("Distance"=w485:dbl, "EncoderDevRef"=w473:T3)  [unwired: 5 in, 4 out]
                n178 = call <vilib>:"WPI_EncoderGet.vi"("EncoderDevRef"=w474) -> ("Distance"=w484:dbl, "EncoderDevRef"=w472:T3)  [unwired: 5 in, 4 out]
                n179 = Greater?(x=w468, y=200) -> (0:w464:bool)
                n180 = Greater?(x=w490, y=0.45) -> (0:w466:bool)
                n181 = Add(x=w485, y=w484) -> (x+y=w483:dbl)
                n182 = Or(x=w466, y=w464) -> (x .or. y?=w465:bool)
                n183 = Greater Or Equal?(x=w483, y=220.0) -> (x >= y?=w476:bool)
                n184 = And(x=w465, y=w476) -> (x .and. y?=w477:bool)
                n185 = Select(t=0.0, s=w465, f=0.75) -> (s? t:f=w486:dbl)
                n186 = Select(t=0.0, s=w476, f=-0.6) -> (s? t:f=w478:dbl)
                n187 = global write "Robot Global Data.vi" "Lift auto"(w486) -> ()
                n188 = call-poly <vilib>:"WPI_RobotDriveArcadeDrive.vi"("Y axis value"=w478, "X axis value"=0.0, "RobotDriveDevRef"=w469) -> ("RobotDriveDevRef"=w471:T11)  [unwired: 6 in, 2 out]
              }
            }
            frame #2 {
              n189 = while {
                tunnel: w493 -> [w498]
                tunnel: w492 -> [w495]
                tunnel: [w494] -> w491
                stop <- w499 stop-if-true
                n190 = call <vilib>:"ADI_IMU_ADIS16448_Get Angles.vi"("ADI IMU DevRef"=w498) -> ("IMU Angles Out"=w502:T17)  [unwired: 7 in, 3 out]
                n191 = call-poly <vilib>:"WPI_RobotDriveArcadeDrive.vi"("Y axis value"=0.0, "X axis value"=0.7, "RobotDriveDevRef"=w495) -> ("RobotDriveDevRef"=w494:T11)  [unwired: 6 in, 2 out]
                n192 = Unbundle(w502) -> ("Z Angle"=w501:dbl)  [unwired: 2 out]
                n193 = Greater Or Equal?(x=w501, y=42.0) -> (x >= y?=w499:bool)
              }
            }
            frame #3 {
              n194 = call-poly <vilib>:"WPI_RobotDriveArcadeDrive.vi"("Y axis value"=-0.6, "X axis value"=0.0, "RobotDriveDevRef"=w507) -> ("RobotDriveDevRef"=w504:T11)  [unwired: 6 in, 2 out]
              n195 = call <vilib>:"WPI_RobotDriveDelayAndUpdateSafety.vi"("Delay (s)"=0.75, "RobotDriveDevRef"=w504) -> ()  [unwired: 8 in, 2 out]
            }
            frame #4 {
              n196 = global write "Robot Global Data.vi" "Pince auto"(FALSE ("Pince auto")) -> ()
            }
          }
        }
        frame 2 {
          # "Scale"
          n197 = flat-sequence {
            tunnel: [w531] -> w523
            tunnel: [w530] -> w522
            tunnel: [w529] -> w521
            tunnel: w515 -> [w528]
            tunnel: w514 -> [w527]
            tunnel: w513 -> [w526]
            tunnel: [w525] -> w512
            tunnel: w511 -> [w525]
            tunnel: [w524] -> w510
            tunnel: w509 -> [w524]
            tunnel: w523 -> [w541]
            tunnel: w522 -> [w540]
            tunnel: [w539] -> w520
            tunnel: w521 -> [w538]
            tunnel: [w538] -> w519
            tunnel: [w537] -> w518
            tunnel: [w536] -> w517
            tunnel: [w535] -> w516
            tunnel: w512 -> [w534]
            tunnel: w510 -> [w533]
            tunnel: w520 -> [w571]
            tunnel: w519 -> [w570]
            tunnel: w518 -> [_]
            tunnel: w517 -> [_]
            tunnel: w516 -> [_]
            frame #0 {
              n198 = global write "Robot Global Data.vi" "Pince auto"(TRUE ("Pince auto")) -> ()
              n199 = call <vilib>:"WPI_EncoderReset.vi"("EncoderDevRef"=w528) -> ("EncoderDevRef"=w531:T3)  [unwired: 9 in, 1 out]
              n200 = call <vilib>:"WPI_EncoderReset.vi"("EncoderDevRef"=w527) -> ("EncoderDevRef"=w530:T3)  [unwired: 9 in, 1 out]
              n201 = call <vilib>:"ADI_IMU_ADIS16448_Reset.vi"("ADI IMU DevRef"=w526) -> ("ADI IMU DevRef Out"=w529:T7)  [unwired: 9 in, 1 out]
            }
            frame #1 {
              n202 = while {
                tunnel: [w554] -> w536
                tunnel: [w553] -> w535
                tunnel: [w552] -> w539
                tunnel: w541 -> [w551]
                tunnel: w540 -> [w550]
                tunnel: [w549] -> w537
                tunnel: w534 -> [w548]
                tunnel: w533 -> [w547]
                i -> [w543]
                stop <- w556 stop-if-true
                n203 = call <vilib>:"WPI_PotentiometerGetNormalized.vi"("PotDevRef"=w548) -> ("Normalized Value"=w569:dbl, "PotDevRef"=w549:T9)  [unwired: 8 in, 1 out]
                n204 = call <vilib>:"WPI_EncoderGet.vi"("EncoderDevRef"=w551) -> ("Distance"=w564:dbl, "EncoderDevRef"=w554:T3)  [unwired: 5 in, 4 out]
                n205 = call <vilib>:"WPI_EncoderGet.vi"("EncoderDevRef"=w550) -> ("Distance"=w563:dbl, "EncoderDevRef"=w553:T3)  [unwired: 5 in, 4 out]
                n206 = Greater?(x=w543, y=370) -> (0:w544:bool)
                n207 = Greater?(x=w569, y=0.47) -> (0:w546:bool)
                n208 = Add(x=w564, y=w563) -> (x+y=w562:dbl)
                n209 = Or(x=w546, y=w544) -> (x .or. y?=w545:bool)
                n210 = Greater Or Equal?(x=w562, y=450.0) -> (x >= y?=w555:bool)
                n211 = And(x=w545, y=w555) -> (x .and. y?=w556:bool)
                n212 = Select(t=0.0, s=w545, f=0.75) -> (s? t:f=w565:dbl)
                n213 = Select(t=0.0, s=w555, f=-0.6) -> (s? t:f=w557:dbl)
                n214 = global write "Robot Global Data.vi" "Lift auto"(w565) -> ()
                n215 = call-poly <vilib>:"WPI_RobotDriveArcadeDrive.vi"("Y axis value"=w557, "X axis value"=0.0, "RobotDriveDevRef"=w547) -> ("RobotDriveDevRef"=w552:T11)  [unwired: 6 in, 2 out]
              }
            }
            frame #2 {
              n216 = while {
                tunnel: w571 -> [w574]
                tunnel: w570 -> [w573]
                tunnel: [w572] -> _
                stop <- w577 stop-if-true
                n217 = call <vilib>:"ADI_IMU_ADIS16448_Get Angles.vi"("ADI IMU DevRef"=w573) -> ("IMU Angles Out"=w580:T17)  [unwired: 7 in, 3 out]
                n218 = Unbundle(w580) -> ("Z Angle"=w579:dbl)  [unwired: 2 out]
                n219 = call-poly <vilib>:"WPI_RobotDriveArcadeDrive.vi"("Y axis value"=0.0, "X axis value"=0.65, "RobotDriveDevRef"=w574) -> ("RobotDriveDevRef"=w572:T11)  [unwired: 6 in, 2 out]
                n220 = Greater?(x=w579, y=20.0) -> (0:w577:bool)
              }
            }
          }
        }
      }
    }
    frame 2 {
      # "Switch=1 Scale=2 Rien=0"
      # "Scale"
      # "Switch"
      # "Right"
      n221 = Not(x=w597) -> (.not. x?=w582:bool)
      n222 = Not(x=w596) -> (.not. x?=w585:bool)
      n223 = Not(x=w607) -> (.not. x?=w581:bool)
      n224 = Not Equal To 0?(x=w606) -> (x != 0?=w605:bool)
      n225 = Equal To 0?(x=w606) -> (x = 0?=w609:bool)
      n226 = Not(x=w582) -> (.not. x?=w610:bool)
      n227 = Or(x=w607, y=w605) -> (x .or. y?=w584:bool)
      n228 = Compound Arithmetic op=AND(w581, w609, w585) -> (w612:bool)
      n229 = Compound Arithmetic op=AND(w581, w585, w610) -> (w611:bool)
      n230 = Compound Arithmetic op=AND(w584, w582) -> (w608:bool)
      n231 = And(x=w581, y=w582) -> (x .and. y?=w583:bool)
      n232 = Compound Arithmetic op=OR(w608, w583) -> (w602:bool)
      n233 = Compound Arithmetic op=OR(w612, w611) -> (w604:bool)
      n234 = Select(t=2.0, s=w602, f=0.0) -> (s? t:f=w600:dbl)
      n235 = Select(t=1.0, s=w604, f=w600) -> (s? t:f=w598:dbl)
      n236 = call <vilib>:"WPI_RobotDriveRefNum Registry Get.vi"("refnum name"="Left and Right Motors") -> ("RobotDriveDevRef"=w586:T11)  [unwired: 9 in, 1 out]
      n237 = call <vilib>:"ADI_IMU_ADIS16448_RefNum Registry Get.vi"("refnum name"="IMU") -> ("ADI IMU DevRef"=w588:T7)  [unwired: 9 in, 1 out]
      n238 = call <vilib>:"WPI_PotentiometerRefNum Registry Get.vi"("refnum name"="Potentiometre") -> ("PotDevRef"=w587:T9)  [unwired: 9 in, 1 out]
      n239 = call <vilib>:"WPI_EncoderRefNum Registry Get.vi"("refnum name"="Right") -> ("EncoderDevRef"=w589:T3)  [unwired: 9 in, 1 out]
      n240 = call <vilib>:"WPI_EncoderRefNum Registry Get.vi"("refnum name"="Left") -> ("EncoderDevRef"=w590:T3)  [unwired: 9 in, 1 out]
      n241 = case shown="1" w598 {
        tunnel: w590 -> [w619 w673 w752]
        tunnel: w589 -> [w618 w672 w751]
        tunnel: w588 -> [w617 w670 w750]
        tunnel: w587 -> [w616 w671 w748]
        tunnel: w586 -> [w614 w669 w746]
        frame 0, Default {
          # "avance"
          # "Avance"
          n242 = flat-sequence {
            tunnel: w617 -> [w629]
            tunnel: w618 -> [w628]
            tunnel: w619 -> [w627]
            tunnel: w616 -> [w623]
            tunnel: [w626] -> w621
            tunnel: [w625] -> w620
            tunnel: [w623] -> w615
            tunnel: w614 -> [w622]
            tunnel: [w622] -> w613
            tunnel: w621 -> [w630]
            tunnel: w620 -> [w631]
            tunnel: w615 -> [w633]
            tunnel: w613 -> [w632]
            frame #0 {
              n243 = call <vilib>:"WPI_EncoderReset.vi"("EncoderDevRef"=w627) -> ("EncoderDevRef"=w626:T3)  [unwired: 9 in, 1 out]
              n244 = call <vilib>:"WPI_EncoderReset.vi"("EncoderDevRef"=w628) -> ("EncoderDevRef"=w625:T3)  [unwired: 9 in, 1 out]
              n245 = call <vilib>:"ADI_IMU_ADIS16448_Reset.vi"("ADI IMU DevRef"=w629) -> ()  [unwired: 9 in, 2 out]
              n246 = global write "Robot Global Data.vi" "Pince auto"(TRUE ("Pince auto")) -> ()
            }
            frame #1 {
              n247 = while {
                tunnel: w633 -> [w657]
                tunnel: w630 -> [w656]
                tunnel: w631 -> [w655]
                tunnel: w632 -> [w654]
                i -> [w635]
                stop <- FALSE stop-if-true
                n248 = call <vilib>:"WPI_PotentiometerGetNormalized.vi"("PotDevRef"=w657) -> ("Normalized Value"=w644:dbl)  [unwired: 8 in, 2 out]
                n249 = call <vilib>:"WPI_EncoderGet.vi"("EncoderDevRef"=w655) -> ("Distance"=w652:dbl)  [unwired: 5 in, 5 out]
                n250 = call <vilib>:"WPI_EncoderGet.vi"("EncoderDevRef"=w656) -> ("Distance"=w653:dbl)  [unwired: 5 in, 5 out]
                n251 = Add(x=w653, y=w652) -> (x+y=w651:dbl)
                n252 = Greater?(x=w644, y=0.3) -> (0:w641:bool)
                n253 = Greater?(x=w635, y=200) -> (0:w642:bool)
                n254 = Or(x=w641, y=w642) -> (x .or. y?=w640:bool)
                n255 = Greater Or Equal?(x=w651, y=255.0) -> (x >= y?=w648:bool)
                n256 = Select(t=0.0 ("Lift auto"), s=w640, f=0.75 ("Lift auto")) -> (s? t:f=w638:dbl)
                n257 = Select(t=0.0, s=w648, f=-0.5 ("Y axis value")) -> (s? t:f=w646:dbl)
                n258 = global write "Robot Global Data.vi" "Lift auto"(w638) -> ()
                n259 = call-poly <vilib>:"WPI_RobotDriveArcadeDrive.vi"("Y axis value"=w646, "X axis value"=0.0, "RobotDriveDevRef"=w654) -> ()  [unwired: 6 in, 3 out]
              }
            }
          }
        }
        frame 1 {
          # "Switch"
          n260 = flat-sequence {
            tunnel: [w685] -> w668
            tunnel: [w684] -> w666
            tunnel: [w683] -> w664
            tunnel: w673 -> [w682]
            tunnel: w672 -> [w681]
            tunnel: w670 -> [w680]
            tunnel: [w679] -> w662
            tunnel: w671 -> [w679]
            tunnel: [w678] -> w660
            tunnel: w669 -> [w678]
            tunnel: w668 -> [w692]
            tunnel: [w692] -> w667
            tunnel: w666 -> [w691]
            tunnel: [w691] -> w665
            tunnel: w664 -> [w690]
            tunnel: [w690] -> w663
            tunnel: w662 -> [w689]
            tunnel: [w689] -> w661
            tunnel: w660 -> [w688]
            tunnel: [w688] -> w659
            tunnel: w667 -> [w700]
            tunnel: w665 -> [w699]
            tunnel: [w698] -> w677
            tunnel: w663 -> [w698]
            tunnel: [w697] -> w676
            tunnel: [w696] -> w675
            tunnel: [w695] -> w674
            tunnel: w661 -> [w694]
            tunnel: w659 -> [w693]
            tunnel: w677 -> [w730]
            tunnel: w676 -> [w729]
            tunnel: w675 -> [_]
            tunnel: w674 -> [_]
            tunnel: [w728] -> w658
            tunnel: w658 -> [w744]
            frame #0 {
              n261 = global write "Robot Global Data.vi" "Pince auto"(TRUE ("Pince auto")) -> ()
              n262 = call <vilib>:"ADI_IMU_ADIS16448_Reset.vi"("ADI IMU DevRef"=w680) -> ("ADI IMU DevRef Out"=w683:T7)  [unwired: 9 in, 1 out]
              n263 = call <vilib>:"WPI_EncoderReset.vi"("EncoderDevRef"=w682) -> ("EncoderDevRef"=w685:T3)  [unwired: 9 in, 1 out]
              n264 = call <vilib>:"WPI_EncoderReset.vi"("EncoderDevRef"=w681) -> ("EncoderDevRef"=w684:T3)  [unwired: 9 in, 1 out]
            }
            frame #1 {
              n265 = Wait (ms)(milliseconds to wait=u32 5) -> ()  [unwired: 1 out]
            }
            frame #2 {
              n266 = while {
                tunnel: w700 -> [w712]
                tunnel: w699 -> [w711]
                tunnel: [w710] -> w696
                tunnel: [w709] -> w695
                tunnel: [w708] -> w697
                tunnel: w694 -> [w707]
                tunnel: w693 -> [w706]
                i -> [w702]
                stop <- w714 stop-if-true
                n267 = call <vilib>:"WPI_PotentiometerGetNormalized.vi"("PotDevRef"=w707) -> ("Normalized Value"=w727:dbl)  [unwired: 8 in, 2 out]
                n268 = call <vilib>:"WPI_EncoderGet.vi"("EncoderDevRef"=w712) -> ("Distance"=w722:dbl, "EncoderDevRef"=w710:T3)  [unwired: 5 in, 4 out]
                n269 = call <vilib>:"WPI_EncoderGet.vi"("EncoderDevRef"=w711) -> ("Distance"=w721:dbl, "EncoderDevRef"=w709:T3)  [unwired: 5 in, 4 out]
                n270 = Greater?(x=w702, y=200) -> (0:w703:bool)
                n271 = Greater?(x=w727, y=0.5) -> (0:w704:bool)
                n272 = Add(x=w722, y=w721) -> (x+y=w720:dbl)
                n273 = Or(x=w704, y=w703) -> (x .or. y?=w705:bool)
                n274 = Greater Or Equal?(x=w720, y=230.0) -> (x >= y?=w713:bool)
                n275 = And(x=w705, y=w713) -> (x .and. y?=w714:bool)
                n276 = Select(t=0.0, s=w705, f=0.75) -> (s? t:f=w723:dbl)
                n277 = Select(t=0.0, s=w713, f=-0.6) -> (s? t:f=w715:dbl)
                n278 = global write "Robot Global Data.vi" "Lift auto"(w723) -> ()
                n279 = call-poly <vilib>:"WPI_RobotDriveArcadeDrive.vi"("Y axis value"=w715, "X axis value"=0.0, "RobotDriveDevRef"=w706) -> ("RobotDriveDevRef"=w708:T11)  [unwired: 6 in, 2 out]
              }
            }
            frame #3 {
              n280 = while {
                tunnel: w730 -> [w735]
                tunnel: w729 -> [w732]
                tunnel: [w731] -> w728
                stop <- w736 stop-if-true
                n281 = call <vilib>:"ADI_IMU_ADIS16448_Get Angles.vi"("ADI IMU DevRef"=w735) -> ("IMU Angles Out"=w739:T17)  [unwired: 7 in, 3 out]
                n282 = call-poly <vilib>:"WPI_RobotDriveArcadeDrive.vi"("Y axis value"=0.0, "X axis value"=-0.65, "RobotDriveDevRef"=w732) -> ("RobotDriveDevRef"=w731:T11)  [unwired: 6 in, 2 out]
                n283 = Unbundle(w739) -> ("Z Angle"=w738:dbl)  [unwired: 2 out]
                n284 = Less Or Equal?(x=w738, y=-42.0) -> (x <= y?=w736:bool)
              }
            }
            frame #4 {
              n285 = call-poly <vilib>:"WPI_RobotDriveArcadeDrive.vi"("Y axis value"=-0.6, "X axis value"=0.0, "RobotDriveDevRef"=w744) -> ("RobotDriveDevRef"=w740:T11)  [unwired: 6 in, 2 out]
              n286 = call <vilib>:"WPI_RobotDriveDelayAndUpdateSafety.vi"("Delay (s)"=1.0, "RobotDriveDevRef"=w740) -> ()  [unwired: 8 in, 2 out]
            }
            frame #5 {
              n287 = global write "Robot Global Data.vi" "Pince auto"(FALSE ("Pince auto")) -> ()
            }
          }
        }
        frame 2 {
          # "Scale"
          n288 = flat-sequence {
            tunnel: [w768] -> w760
            tunnel: [w767] -> w759
            tunnel: [w766] -> w758
            tunnel: w752 -> [w765]
            tunnel: w751 -> [w764]
            tunnel: w750 -> [w763]
            tunnel: [w762] -> w749
            tunnel: w748 -> [w762]
            tunnel: [w761] -> w747
            tunnel: w746 -> [w761]
            tunnel: w760 -> [w778]
            tunnel: w759 -> [w777]
            tunnel: [w776] -> w757
            tunnel: w758 -> [w775]
            tunnel: [w775] -> w756
            tunnel: [w774] -> w755
            tunnel: [w773] -> w754
            tunnel: [w772] -> w753
            tunnel: w749 -> [w771]
            tunnel: w747 -> [w770]
            tunnel: w757 -> [w808]
            tunnel: w756 -> [w807]
            tunnel: w755 -> [_]
            tunnel: w754 -> [_]
            tunnel: w753 -> [_]
            frame #0 {
              n289 = global write "Robot Global Data.vi" "Pince auto"(TRUE ("Pince auto")) -> ()
              n290 = call <vilib>:"WPI_EncoderReset.vi"("EncoderDevRef"=w765) -> ("EncoderDevRef"=w768:T3)  [unwired: 9 in, 1 out]
              n291 = call <vilib>:"WPI_EncoderReset.vi"("EncoderDevRef"=w764) -> ("EncoderDevRef"=w767:T3)  [unwired: 9 in, 1 out]
              n292 = call <vilib>:"ADI_IMU_ADIS16448_Reset.vi"("ADI IMU DevRef"=w763) -> ("ADI IMU DevRef Out"=w766:T7)  [unwired: 9 in, 1 out]
            }
            frame #1 {
              n293 = while {
                tunnel: [w791] -> w773
                tunnel: [w790] -> w772
                tunnel: [w789] -> w776
                tunnel: w778 -> [w788]
                tunnel: w777 -> [w787]
                tunnel: [w786] -> w774
                tunnel: w771 -> [w785]
                tunnel: w770 -> [w784]
                i -> [w783]
                stop <- w793 stop-if-true
                n294 = call <vilib>:"WPI_PotentiometerGetNormalized.vi"("PotDevRef"=w785) -> ("Normalized Value"=w806:dbl, "PotDevRef"=w786:T9)  [unwired: 8 in, 1 out]
                n295 = call <vilib>:"WPI_EncoderGet.vi"("EncoderDevRef"=w788) -> ("Distance"=w801:dbl, "EncoderDevRef"=w791:T3)  [unwired: 5 in, 4 out]
                n296 = call <vilib>:"WPI_EncoderGet.vi"("EncoderDevRef"=w787) -> ("Distance"=w800:dbl, "EncoderDevRef"=w790:T3)  [unwired: 5 in, 4 out]
                n297 = Greater?(x=w783, y=370) -> (0:w779:bool)
                n298 = Greater?(x=w806, y=0.47) -> (0:w781:bool)
                n299 = Add(x=w801, y=w800) -> (x+y=w799:dbl)
                n300 = Or(x=w781, y=w779) -> (x .or. y?=w780:bool)
                n301 = Greater Or Equal?(x=w799, y=450.0) -> (x >= y?=w792:bool)
                n302 = And(x=w780, y=w792) -> (x .and. y?=w793:bool)
                n303 = Select(t=0.0, s=w780, f=0.75) -> (s? t:f=w802:dbl)
                n304 = Select(t=0.0, s=w792, f=-0.6) -> (s? t:f=w794:dbl)
                n305 = global write "Robot Global Data.vi" "Lift auto"(w802) -> ()
                n306 = call-poly <vilib>:"WPI_RobotDriveArcadeDrive.vi"("Y axis value"=w794, "X axis value"=0.0, "RobotDriveDevRef"=w784) -> ("RobotDriveDevRef"=w789:T11)  [unwired: 6 in, 2 out]
              }
            }
            frame #2 {
              n307 = while {
                tunnel: w808 -> [w811]
                tunnel: w807 -> [w810]
                tunnel: [w809] -> _
                stop <- w814 stop-if-true
                n308 = call <vilib>:"ADI_IMU_ADIS16448_Get Angles.vi"("ADI IMU DevRef"=w810) -> ("IMU Angles Out"=w817:T17)  [unwired: 7 in, 3 out]
                n309 = Unbundle(w817) -> ("Z Angle"=w816:dbl)  [unwired: 2 out]
                n310 = call-poly <vilib>:"WPI_RobotDriveArcadeDrive.vi"("Y axis value"=0.0, "X axis value"=-0.65, "RobotDriveDevRef"=w811) -> ("RobotDriveDevRef"=w809:T11)  [unwired: 6 in, 2 out]
                n311 = Less?(x=w816, y=-20.0) -> (x < y?=w814:bool)
              }
            }
          }
        }
      }
    }
  }
